vi "题目四.vi"() -> ()   [LabVIEW 2017]
uses:
  <vilib>/measure/NI_MABase.lvlib
panel:
  out "error out":errorcluster caption="错误输出"
  out "最小值":dbl
  out "Y":dbl[](array[numeric])
  out "dt":dbl
  out "signal out":waveform(dbl) caption="信号输出"
  in  "error in (no error)":errorcluster caption="错误输入（无错误）"
  in  "reset signal":bool caption="重置信号"
  in  "sampling info":cluster{"Fs":dbl, "#s":dbl}={"Fs"=1000.0, "#s"=1000.0} caption="采样信息" {"Fs" format="%.2p"}
  in  "相位":dbl caption="相位输入" format="%0.2f"
  in  "频率":dbl=0.0078125 format="%0.4e"
  in  "幅值":dbl=1.0 format="%0.2f"
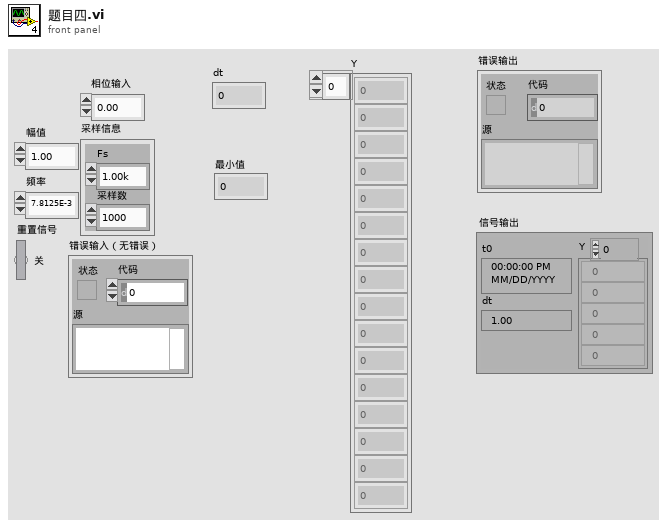
[diagram p1: front panel]
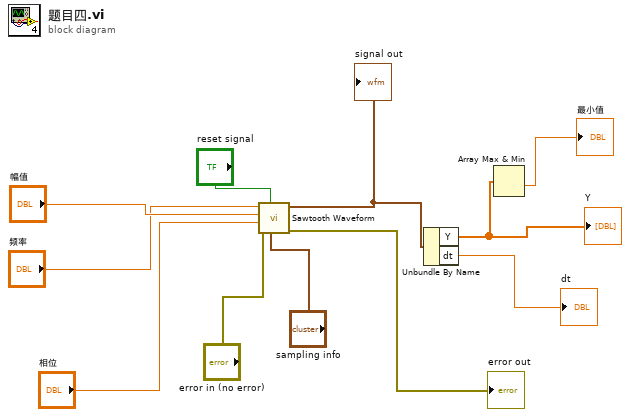
[diagram p0: block diagram]
diagram:
  n1 = call <vilib>:"Sawtooth Waveform.vi"("sampling info"="sampling info", "reset signal"="reset signal", "error in (no error)"="error in (no error)", "phase"="相位", "amplitude"="幅值", "frequency"="频率") -> ("error out"=→"error out":errorcluster, "signal out"=w5:waveform(dbl))  [unwired: 4 in]
  "signal out" <- w5
  n2 = Unbundle By Name(w5) -> ("Y"=w3:dbl[], "dt"=→"dt":dbl)
  "Y" <- w3
  n3 = Array Max & Min(array=w3) -> (min value=→"最小值":dbl)  [unwired: 3 out]
